vi "TiePie.Scp.ScpGetConnectionTestData.vi"(8 "error in (no error)":errorcluster, 9 "wChannelCount":u16, 10 "pBuffer":i8, 11 "GenHandle":T1) -> (3 "GenHandle out":T1)   [LabVIEW 2013, in "LVTiePie.lvlib"]
uses:
  LVTiePie.lvlib
  PAN/LabVEW/Tie Pie/bin/libtiepie.dll
  TiePie.Gen.handle.ctl
panel:
  out "return type":u16
  out "error out":errorcluster
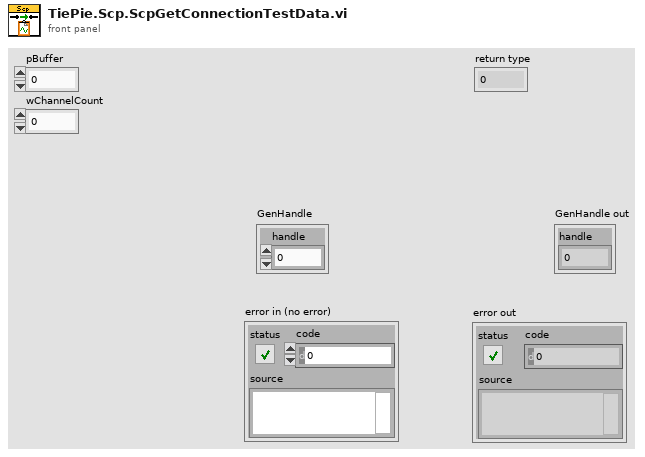
[diagram p1: front panel]
types:
  T1 = typedef "TiePie.Gen.handle.ctl" = cluster{"handle":u32}
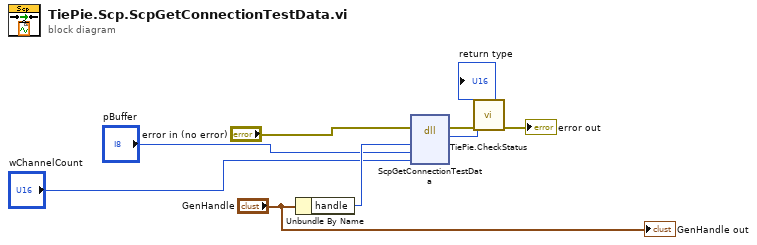
[diagram p0: block diagram]
diagram:
  n1 = Unbundle By Name("GenHandle") -> ("handle"=w7:u32)
  n2 = dll-call lib="C:/Users/mbirski/Desktop/PAN/LabVEW/Tie Pie/bin/libtiepie.dll" fn="ScpGetConnectionTestData"(error in="error in (no error)", "handle"=w7, "pBuffer"="pBuffer", "wChannelCount"="wChannelCount") -> (error out=w5:errorcluster, "numberOfElements"=→"return type":u16)  [unwired: 5 in, 1 out]
  n3 = call "TiePie.CheckStatus.vi"("error in (no error)"=w5) -> ("error out"=→"error out":errorcluster)  [unwired: 10 in]
  "GenHandle out" <- "GenHandle"
